vi "PID Structure Conversion (DBL Array).vi"(4 "derivative unit":T2 items=["min", "s"], 5 "proportional unit":T4 items=["Gain (K)", "Band (PB)"], 6 "integral unit":T2 items=["min", "s"], 7 "PID structure":T3 items=["Academic (Standard)", "Parallel", "Series"], 9 "derivative":dbl[](array[numeric]), 10 "integral":dbl[](array[numeric]), 11 "proportional":dbl[](array[numeric])) -> (3 "PID parameters":T1(array[cluster]))   [LabVIEW 2020, in "NI_PID_pid.lvlib"]
doc: "Converts a PID controller or controllers in Academic, Parallel, or Series form into the form (Academic) and <B>PID gains</B> units that the PID VIs expect. Wire data to the <B>proportional</B>, <B>integral</B>, or <B>derivative</B> input to determine the polymorphic instance to use, or manually select the instance."
uses:
  <vilib>/addons/control/pid/NI_PID_pid.lvlib
  <vilib>/addons/control/pid/pid.llb/PID Gain Unit.ctl
  <vilib>/addons/control/pid/pid.llb/PID Structure.ctl
  <vilib>/addons/control/pid/pid.llb/PID Time Unit.ctl
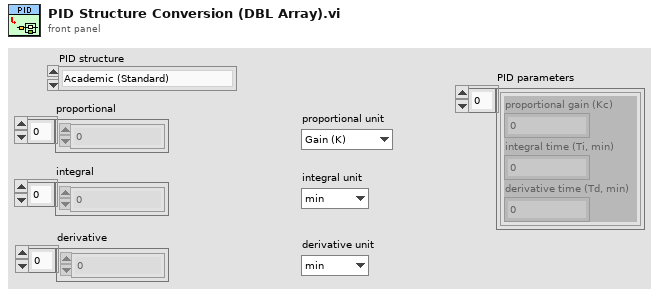
[diagram p1: front panel]
types:
  T1 = cluster{"proportional gain (Kc)":dbl, "integral time (Ti, min)":dbl, "derivative time (Td, min)":dbl}[]
  T2 = typedef "NI_PID_pid.lvlib/PID Time Unit.ctl" = u16
  T3 = typedef "NI_PID_pid.lvlib/PID Structure.ctl" = u16
  T4 = typedef "NI_PID_pid.lvlib/PID Gain Unit.ctl" = u16
  T5 = cluster{"proportional gain (Kc)":dbl, "integral time (Ti, min)":dbl, "derivative time (Td, min)":dbl}
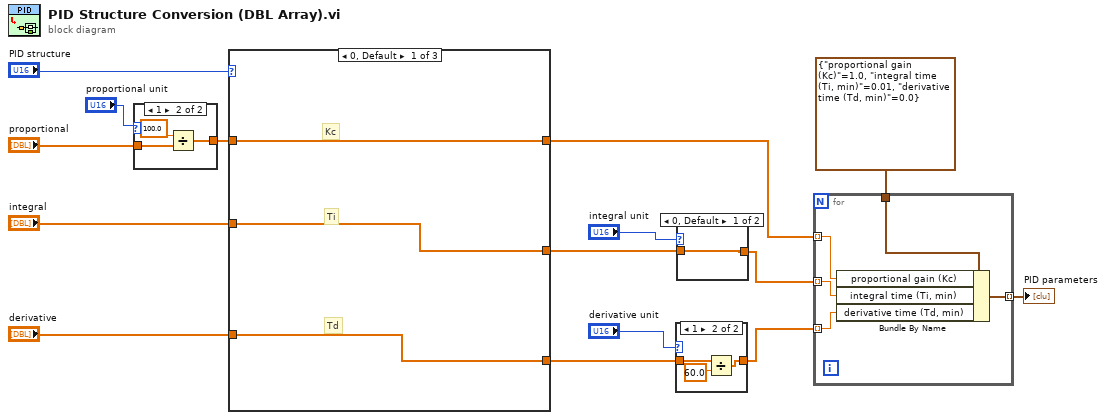
[diagram p0: block diagram]
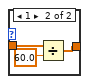
[diagram p4: hidden frame]
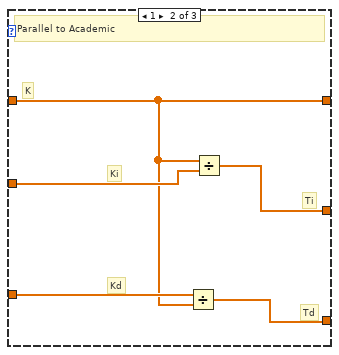
[diagram p5: hidden frame]
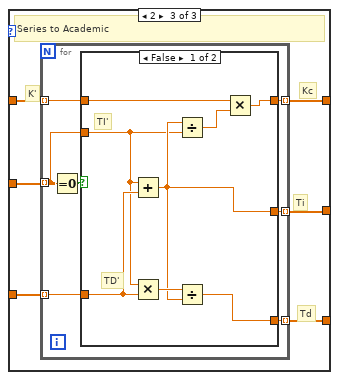
[diagram p6: hidden frame]
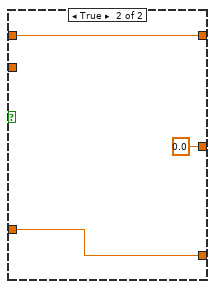
[diagram p7: hidden frame]
diagram:
  n1 = case shown="1" "proportional unit" {
    tunnel: "proportional" -> [w16 w17]
    tunnel: [w16 w19] -> w6
    frame 0, Default {
    }
    frame 1 {
      n2 = Divide(x=100.0, y=w17) -> (x/y=w19:dbl[])
    }
  }
  n3 = case shown="0, Default" "PID structure" {
    tunnel: "derivative" -> [w22 w25 w31]
    tunnel: "integral" -> [w21 w27 w28]
    tunnel: [w22 w23 w29] -> w10
    tunnel: [w21 w26 w30] -> w9
    tunnel: [w20 w24 w32] -> w5
    tunnel: w6 -> [w20 w24 w33]
    frame 0, Default {
      # "Td"
      # "Ti"
      # "Kc"
    }
    frame 1 {
      # "Td"
      # "Ti"
      # "Kd"
      # "Ki"
      # "K"
      # "Parallel to Academic"
      n4 = Divide(x=w25, y=w24) -> (x/y=w23:dbl[])
      n5 = Divide(x=w24, y=w27) -> (x/y=w26:dbl[])
    }
    frame 2 {
      # "K'"
      # "Td"
      # "Kc"
      # "Ti"
      # "Series to Academic"
      n6 = for {
        tunnel: w33 -> [w40] mode=indexing
        tunnel: [w39] -> w32 mode=indexing
        tunnel: w31 -> [w38] mode=indexing
        tunnel: [w37] -> w30 mode=indexing
        tunnel: [w36] -> w29 mode=indexing
        tunnel: w28 -> [w34] mode=indexing
        n7 = Equal To 0?(x=w34) -> (x = 0?=w35:bool)
        n8 = case shown="False" w35 {
          tunnel: w40 -> [w48 w51]
          tunnel: [w46 w51] -> w39
          tunnel: w38 -> [w45 w49]
          tunnel: [w43 0.0] -> w37
          tunnel: [w42 w49] -> w36
          tunnel: w34 -> [w41 _]
          frame False {
            # "TD'"
            # "TI'"
            n9 = Add(x=w41, y=w45) -> (x+y=w43:dbl)
            n10 = Multiply(x=w41, y=w45) -> (x*y=w44:dbl)
            n11 = Divide(x=w43, y=w41) -> (x/y=w47:dbl)
            n12 = Divide(x=w44, y=w43) -> (x/y=w42:dbl)
            n13 = Multiply(x=w48, y=w47) -> (x*y=w46:dbl)
          }
          frame True {
          }
        }
      }
    }
  }
  n14 = case shown="1" "derivative unit" {
    tunnel: w10 -> [w52 w55]
    tunnel: [w52 w53] -> w3
    frame 0, Default {
    }
    frame 1 {
      n15 = Divide(x=w55, y=60.0) -> (x/y=w53:dbl[])
    }
  }
  n16 = case shown="0, Default" "integral unit" {
    tunnel: w9 -> [w56 w59]
    tunnel: [w56 w57] -> w4
    frame 0, Default {
    }
    frame 1 {
      n17 = Divide(x=w59, y=60.0) -> (x/y=w57:dbl[])
    }
  }
  n18 = for {
    tunnel: w5 -> [w61] mode=indexing
    tunnel: w4 -> [w62] mode=indexing
    tunnel: w3 -> [w63] mode=indexing
    tunnel: T5 {"proportional gain (Kc)"=1.0, "integral time (Ti, min)"=0.01, "derivative time (Td, min)"=0.0} ("PID gains") -> [w64]
    tunnel: [w60] -> w1 mode=indexing
    n19 = Bundle By Name(cluster=w64, "proportional gain (Kc)"=w61, "integral time (Ti, min)"=w62, "derivative time (Td, min)"=w63) -> (w60:T5)
  }
  "PID parameters" <- w1
